vi "string to enum.vi"(8 "error in":errorcluster, 10 "String":string, 11 "Enum":refnum<vi>) -> (0 "error out":errorcluster, 3 "Value":i32)   [LabVIEW 2013, in "Table Manager.lvlib"]
uses:
  Table Manager.lvlib
  <vilib>/NI/Tag Bus/tag/Data Type.ctl
  <vilib>/NI/Tag Bus/tag/tag descriptor.lvclass
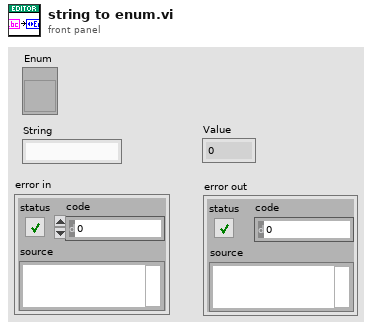
[diagram p1: front panel]
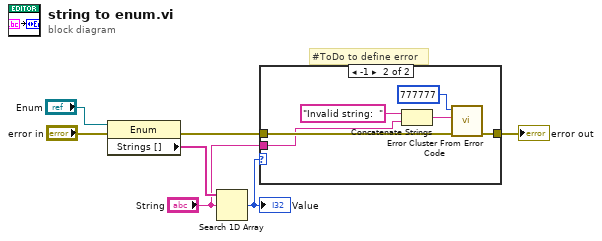
[diagram p0: block diagram]
diagram:
  # "#ToDo to define error"
  n1 = property class="Enum"(reference="Enum", error in="error in") -> (error out=w5:errorcluster, "Strings []"=w3:string[])  [unwired: 1 out]
  n2 = Search 1D Array(1D array=w3, element="String") -> (index of element=w2:i32)  [unwired: 1 in]
  "Value" <- w2
  n3 = case shown="-1" w2 {
    tunnel: w5 -> [w8 w14]
    tunnel: [w8 w13] -> w4
    tunnel: "String" -> [_ w11]
    frame 0, Default {
    }
    frame -1 {
      n4 = Concatenate Strings("Invalid string:  " ("error message (\"\")"), w11) -> (w9:string)
      n5 = call <vilib>:"Error Cluster From Error Code.vi"("error in (no error)"=w14, "error message (\"\")"=w9, "error code (0)"=777777) -> ("error out"=w13:errorcluster)  [unwired: 6 in]
    }
  }
  "error out" <- w4
